vi "After Launch Init Core.vi"(8 "error in (no error)":errorcluster, 11 "CS++IEFWerner in":refnum<class "CS++IEFWerner.lvclass">) -> (0 "error out":errorcluster, 3 "CS++IEFWerner out":refnum<class "CS++IEFWerner.lvclass">)   [LabVIEW 2015, in "CS++IEFWerner.lvlib" / "CS++IEFWerner.lvclass"]
doc: "Use <b>Pre Launch init.vi</b> method for sanity checks that are supposed to prevent the actor from launching if they fail. Use <B>this</B> method instead to initialize this actor when it has been activated. A corresponding high priority message will become dispatched before the <B>Actor Core.vi</b> is called.\n\n<b>Derived classed should call the parent methode first</b> and their own initialization code after.\n\nRefer also to the ongoing discussion at https://decibel.ni.com/content/message/57394#57394."
uses:
  CS++IEFWerner.lvclass
  CS++IEFWerner.lvclass/CS++IEFWerner.ctl
  CSPP_Core/Classes/CS++ProcessVariables/ProcessVariable/PV.lvclass
  CSPP_DSC/Classes/DSCConnection/DSCConnection.lvclass
  CSPP_Core/Classes/CS++ProcessVariables/ProcessVariable/PV.lvclass/PV.ctl
  CSPP_Core/Classes/CS++ProcessVariables/PVConnection/PVConnection.lvclass/PVConnection.ctl
  <vilib>/ActorFramework/Actor/Actor.lvclass/Actor.ctl
  <vilib>/ActorFramework/Message Enqueuer/Message Enqueuer.lvclass/Message Enqueuer.ctl
  CS++IEFWerner Messages/Update_Readback Msg/Update_Readback Msg.lvclass/Update_Readback Msg.ctl
  CSPP_Core/Classes/CS++ProcessVariables/ProcessVariable/Write Name.vi
  CSPP_Core/Classes/CS++ProcessVariables/ProcessVariable/Write PV URL.vi
  <vilib>/ActorFramework/Message Enqueuer/Init from Existing Queue.vi
  <vilib>/ActorFramework/Message Enqueuer/Enqueue.vi
  <vilib>/Utility/error.llb/Error Cluster From Error Code.vi
  <vilib>/ActorFramework/Message Priority Queue/Priority Enqueue.vi
  CSPP_DeviceBase/CS++Motor/CS++Motor.lvclass
  <vilib>/ActorFramework/Message Enqueuer/Message Enqueuer.lvclass
  CS++IEFWerner Messages/Update_Readback Msg/Update_Readback Msg.lvclass
  CSPP_Core/Classes/CS++ProcessVariables/PVConnection/PVConnection.lvclass
  <vilib>/ActorFramework/Actor/Actor.lvclass
  CSPP_Core/Actors/CS++DeviceActor Messages/Reset Device Msg/Reset Device Msg.lvclass
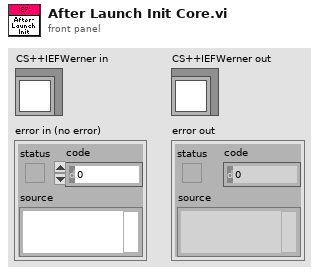
[diagram p1: front panel]
types:
  T1 = cluster{"Read Access":enum8{"Allowed", "Required", "None"}, "Write Access":enum8{"Allowed", "Required", "None"}}
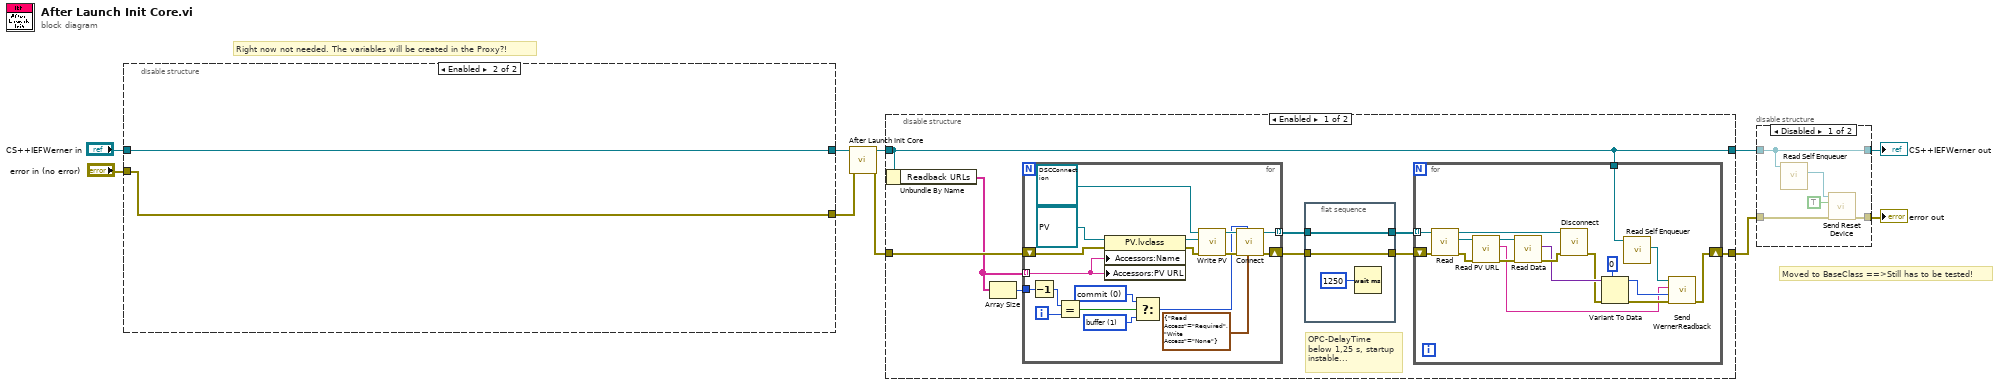
[diagram p0: block diagram]
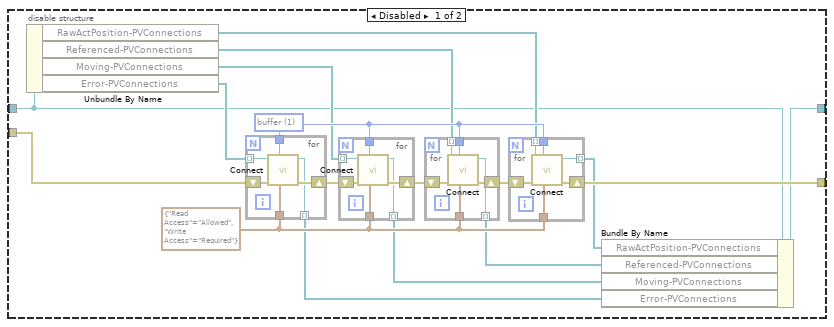
[diagram p4: hidden frame]
diagram:
  # "Moved to BaseClass ==>Still has to be tested!"
  # "Right now not needed. The variables will be created in the Proxy?!"
  n1 = disable-structure shown="Enabled" {
    disable-tunnel: "error in (no error)" -> [w27 w52]
    disable-tunnel: [w21 w52] -> w9
    disable-tunnel: "CS++IEFWerner in" -> [w16 w53]
    disable-tunnel: [w15 w53] -> w7
    frame Disabled {
      w23 = T1 {"Read Access"=enum."Allowed", "Write Access"=enum."Required"} ("Access (R/W allowed)")
      w22 = u16 1 items=["commit", "buffer"] ("Mode (buffer)")
      n2 = Unbundle By Name(w16) -> ("RawActPosition-PVConnections"=w17:refnum<class "PVConnection.lvclass">[], "Referenced-PVConnections"=w18:refnum<class "PVConnection.lvclass">[], "Moving-PVConnections"=w19:refnum<class "PVConnection.lvclass">[], "Error-PVConnections"=w20:refnum<class "PVConnection.lvclass">[])
      n3 = for {
        tunnel: w23 -> [w49]
        tunnel: w22 -> [w48]
        shift-right: [w50] -> w26
        shift-left: w27 -> [w51]
        tunnel: w20 -> [w47] mode=indexing
        tunnel: [w46] -> w14 mode=indexing
        n4 = call "Connect.vi"("Access (R/W allowed)"=w49, "Mode (buffer)"=w48, "Error In"=w51, "PVConnection in"=w47) -> ("Error Out"=w50:errorcluster, "PVConnection out"=w46:refnum<class "PVConnection.lvclass">)  [unwired: 6 in]
      }
      n5 = for {
        tunnel: w23 -> [w43]
        tunnel: w22 -> [w42]
        shift-right: [w44] -> w25
        shift-left: w26 -> [w45]
        tunnel: w19 -> [w41] mode=indexing
        tunnel: [w40] -> w13 mode=indexing
        n6 = call "Connect.vi"("Access (R/W allowed)"=w43, "Mode (buffer)"=w42, "Error In"=w45, "PVConnection in"=w41) -> ("Error Out"=w44:errorcluster, "PVConnection out"=w40:refnum<class "PVConnection.lvclass">)  [unwired: 6 in]
      }
      n7 = for {
        tunnel: w23 -> [w37]
        tunnel: w22 -> [w36]
        shift-right: [w38] -> w24
        shift-left: w25 -> [w39]
        tunnel: w18 -> [w35] mode=indexing
        tunnel: [w34] -> w12 mode=indexing
        n8 = call "Connect.vi"("Access (R/W allowed)"=w37, "Mode (buffer)"=w36, "Error In"=w39, "PVConnection in"=w35) -> ("Error Out"=w38:errorcluster, "PVConnection out"=w34:refnum<class "PVConnection.lvclass">)  [unwired: 6 in]
      }
      n9 = for {
        tunnel: w23 -> [w32]
        tunnel: w22 -> [w31]
        shift-right: [w30] -> w21
        shift-left: w24 -> [w33]
        tunnel: w17 -> [w29] mode=indexing
        tunnel: [w28] -> w11 mode=indexing
        n10 = call "Connect.vi"("Access (R/W allowed)"=w32, "Mode (buffer)"=w31, "Error In"=w33, "PVConnection in"=w29) -> ("Error Out"=w30:errorcluster, "PVConnection out"=w28:refnum<class "PVConnection.lvclass">)  [unwired: 6 in]
      }
      n11 = Bundle By Name(cluster=w16, "RawActPosition-PVConnections"=w11, "Referenced-PVConnections"=w12, "Moving-PVConnections"=w13, "Error-PVConnections"=w14) -> (w15:refnum<class "CS++IEFWerner.lvclass">)
    }
    frame Enabled {
    }
  }
  n12 = call-parent "After Launch Init Core.vi"("error in (no error)"=w9, "CS++Motor in"=w7) -> ("error out"=w6:errorcluster, "CS++Motor out"=w5:refnum<class "CS++IEFWerner.lvclass">)  [unwired: 8 in]
  n13 = disable-structure shown="Enabled" {
    disable-tunnel: w6 -> [w62 w101]
    disable-tunnel: w5 -> [w54 w102]
    disable-tunnel: [w55 w101] -> w3
    disable-tunnel: [w54 w102] -> w2
    frame Enabled {
      # "OPC-DelayTime\nbelow 1,25 s, startup\ninstable..."
      n14 = Unbundle By Name(w54) -> ("Readback URLs"=w61:string[])
      n15 = Array Size(array=w61) -> (size(s)=w60:i32)
      n16 = for {
        tunnel: w61 -> [w94] mode=indexing
        tunnel: w60 -> [w92]
        shift-right: [w85] -> w56
        shift-left: w62 -> [w95]
        tunnel: [w84] -> w58 mode=indexing
        i -> [w93]
        w89 = u16 0 items=["commit", "buffer"] ("Mode (buffer)")
        w88 = u16 1 items=["commit", "buffer"] ("Mode (buffer)")
        n17 = Decrement(x=w92) -> (x-1=w91:i32)
        n18 = Equal?(x=w91, y=w93) -> (x = y?=w90:bool)
        n19 = property class="PV.lvclass"(reference=refnum<class "PV.lvclass"> refnum ("CS++ProcessVariables.lvlib:PV.lvclass"), error in=w95, "Accessors:Name"=w94, "Accessors:PV URL"=w94) -> (reference out=w99:refnum<class "PV.lvclass">, error out=w97:errorcluster)
        n20 = Select(t=w89, s=w90, f=w88) -> (s? t:f=w87:u16)
        n21 = call "Write PV.vi"("error in (no error)"=w97, "PV"=w99, "PVConnection in"=refnum<class "DSCConnection.lvclass"> refnum ("CS++DSCConnection.lvlib:DSCConnection.lvclass")) -> ("error out"=w96:errorcluster, "PVConnection out"=w98:refnum<class "DSCConnection.lvclass">)  [unwired: 7 in]
        n22 = call "Connect.vi"("Access (R/W allowed)"=T1 {"Read Access"=enum."Required", "Write Access"=enum."None"}, "Mode (buffer)"=w87, "Error In"=w96, "PVConnection in"=w98) -> ("Error Out"=w85:errorcluster, "PVConnection out"=w84:refnum<class "DSCConnection.lvclass">)  [unwired: 6 in]
      }
      n23 = flat-sequence {
        tunnel: [w65] -> w59
        tunnel: w58 -> [w65]
        tunnel: [w64] -> w57
        tunnel: w56 -> [w64]
        frame #0 {
          n24 = Wait (ms)(milliseconds to wait=u32 1250) -> ()  [unwired: 1 out]
        }
      }
      n25 = for {
        tunnel: w59 -> [w82] mode=indexing
        tunnel: w54 -> [w74]
        shift-right: [w71] -> w55
        shift-left: w57 -> [w81]
        n26 = call "Read.vi"("error in (no error)"=w81, "PVConnection in"=w82) -> ("error out"=w67:errorcluster, "PV"=w68:refnum<class "PV.lvclass">, "PVConnection out"=w80:refnum<class "DSCConnection.lvclass">)  [unwired: 6 in, 1 out]
        n27 = call "Read PV URL.vi"("error in (no error)"=w67, "PV in"=w68) -> ("error out"=w70:errorcluster, "PV URL"=w66:string, "PV out"=w69:refnum<class "PV.lvclass">)  [unwired: 7 in]
        n28 = call "Read Data.vi"("error in (no error)"=w70, "PV in"=w69) -> ("error out"=w79:errorcluster, "Data"=w77:variant)  [unwired: 7 in, 1 out]
        n29 = call "Disconnect.vi"("error in (no error)"=w79, "PVConnection in"=w80) -> ("error out"=w76:errorcluster)  [unwired: 8 in, 1 out]
        n30 = Variant To Data(error in=w76, type=u32 0, Variant=w77) -> (data=w72:u32, error out=w73:errorcluster)
        n31 = call <vilib>:"Read Self Enqueuer.vi"("Actor"=w74) -> ("Self Enqueuer"=w78:refnum<class "Message Enqueuer.lvclass">)  [unwired: 10 in]
        n32 = call "Send WernerReadback.vi"("error in (no error)"=w73, "Value"=w72, "URL"=w66, "Message Enqueuer"=w78) -> ("error out"=w71:errorcluster)  [unwired: 6 in, 1 out]
      }
    }
    frame Disabled {
    }
  }
  n33 = disable-structure shown="Disabled" {
    disable-tunnel: [w105 w108] -> w4
    disable-tunnel: w3 -> [w104 w108]
    disable-tunnel: w2 -> [w103 w109]
    disable-tunnel: [w103 w109] -> w1
    frame Disabled {
      n34 = call <vilib>:"Read Self Enqueuer.vi"("Actor"=w103) -> ("Self Enqueuer"=w107:refnum<class "Message Enqueuer.lvclass">)  [unwired: 10 in]
      n35 = call "Send Reset Device.vi"("error in (no error)"=w104, "Reset"=TRUE, "Message Enqueuer"=w107) -> ("error out"=w105:errorcluster)  [unwired: 7 in, 1 out]
    }
    frame Enabled {
    }
  }
  "error out" <- w4
  "CS++IEFWerner out" <- w1
